vi "StopProcesses.vi"(8 "error in (no error)":errorcluster, 9 "timeout in ms (-1)":i32=-1, 11 "SMO":refnum<class "SMO.lvclass">) -> (0 "error out":errorcluster, 3 "SMO out":refnum<class "SMO.lvclass">)   [LabVIEW 2013, in "SMO.lvclass"]
doc: "Stops all processes in the JKI SMO.\n\n---------------------------------------------------------------\nJKI State Machine Objects™\nhttp://jki.net/state-machine-objects/\nCopyright (C) 2005-2015, JKI <info@jki.net>\nALL RIGHTS RESERVED"
uses:
  SMO.lvclass
panel:
  # "For instructions on how to use the JKI State Machine Objects, examples and video tutorials, visit:\nhttp://jki.net/state-machine-objects/\n\nJKI State Machine Objects™\nhttp://jki.net/state-machine-objects/\nCopyright (C) 2005-2015, JKI <info@jki.net>\nALL RIGHTS RESERVED"
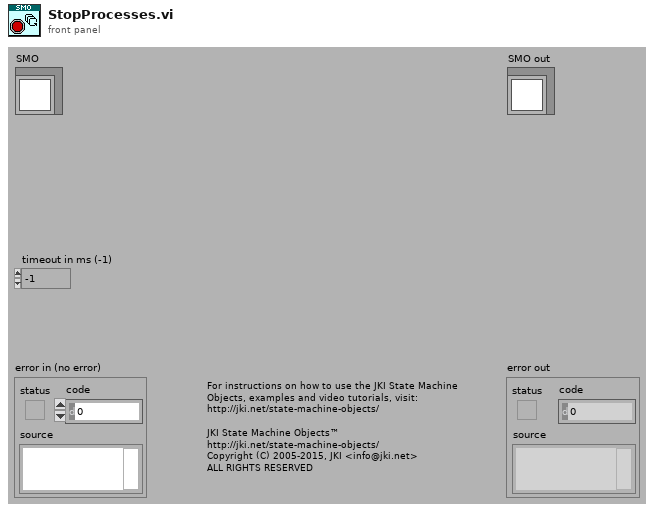
[diagram p1: front panel]
types:
  T1 = typedef "SMO.lvclass/Process Error Notification--Cluster.ctl" = cluster{"error":errorcluster}
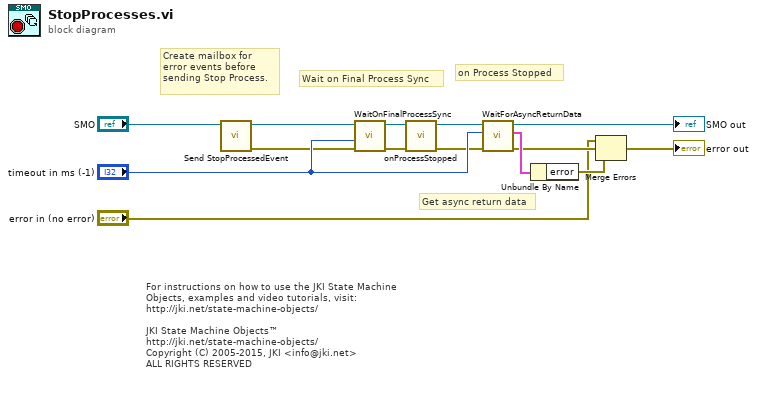
[diagram p0: block diagram]
diagram:
  # "on Process Stopped"
  # "Get async return data"
  # "Wait on Final Process Sync"
  # "Create mailbox for\nerror events before\nsending Stop Process."
  # "For instructions on how to use the JKI State Machine Objects, examples and video tutorials, visit:\nhttp://jki.net/state-machine-objects/\n\nJKI State Machine Objects™\nhttp://jki.net/state-machine-objects/\nCopyright (C) 2005-2015, JKI <info@jki.net>\nALL RIGHTS RESERVED"
  n1 = call "Send StopProcessedEvent.vi"("SMO"="SMO") -> ("error out"=w9:errorcluster, "SMO out"=w10:refnum<class "SMO.lvclass">)  [unwired: 9 in]
  n2 = call "WaitOnFinalProcessSync.vi"("error in (no error)"=w9, "timeout in ms (-1)"="timeout in ms (-1)", "SMO"=w10) -> ("error out"=w2:errorcluster, "SMO out"=w5:refnum<class "SMO.lvclass">)  [unwired: 7 in]
  n3 = call-dynamic "onProcessStopped.vi"("error in (no error)"=w2, "SMO"=w5) -> ("error out"=w3:errorcluster, "SMO out"=w4:refnum<class "SMO.lvclass">)  [unwired: 8 in]
  n4 = call "WaitForAsyncReturnData.vi"("error in (no error)"=w3, "timeout in ms (-1)"="timeout in ms (-1)", "SMO"=w4) -> ("error out"=w6:errorcluster, "Process Notification"=w8:T1, "SMO out"=→"SMO out":refnum<class "SMO.lvclass">)  [unwired: 6 in]
  n5 = Unbundle By Name(w8) -> ("error"=w7:errorcluster)
  n6 = Merge Errors("error in (no error)", w6, w7) -> (→"error out":errorcluster)
